vi "FlattenXMLData.vi"() -> ()   [LabVIEW 2020]
uses:
  <vilib>/Utility/xml.llb/Write to XML File.vi
panel:
  out "XML Output":string
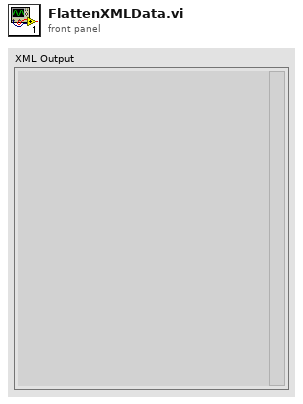
[diagram p1: front panel]
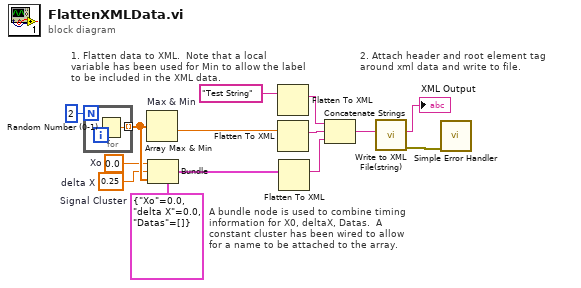
[diagram p0: block diagram]
diagram:
  w8 = cluster{"Xo":dbl, "delta X":dbl, "Datas":dbl[]} {"Xo"=0.0, "delta X"=0.0, "Datas"=[]}  # Signal Cluster
  w13 = 0.25  # delta X
  w12 = 0.0  # Xo
  # "A bundle node is used to combine timing information for X0, deltaX, Datas.  A constant cluster has been wired to allow for a name to be attached to the array."
  # "2. Attach header and root element tag around xml data and write to file."
  # "1. Flatten data to XML.  Note that a local variable has been used for Min to allow the label to be included in the XML data."
  n1 = for {
    N: 2 -> [_]
    tunnel: [w15] -> w14 mode=indexing
    n2 = Random Number (0-1)() -> (number: 0 to 1=w15:dbl)
  }
  n3 = Array Max & Min "Max & Min"(array=w14) -> (min value=w3:dbl)  [unwired: 3 out]
  n4 = Bundle(cluster=w8, "Xo"=w12, "delta X"=w13, "Datas"=w14) -> (w11:cluster{"Xo":dbl, "delta X":dbl, "Datas":dbl[]})
  n5 = Flatten To XML(6:"Test String") -> (2:w2:string)
  n6 = Flatten To XML(6:w3) -> (2:w9:string)
  n7 = Flatten To XML(6:w11) -> (2:w10:string)
  n8 = Concatenate Strings(w2, w9, w10) -> (w7:string)
  n9 = call-poly <vilib>:"Write to XML File(string).vi"("XML Input"=w7) -> ("error out"=w5:errorcluster, "XML String"=→"XML Output":string)  [unwired: 4 in, 5 out]
  n10 = call <vilib>:"Simple Error Handler.vi"("error in (no error)"=w5) -> ()  [unwired: 1 in, 8 out]
